vi "Read Loop order.vi"(11 "Toggle 8 in":refnum<class "Toggle 8.lvclass">) -> (2 "Loop order":bool, 3 "Toggle 8 out":refnum<class "Toggle 8.lvclass">)   [LabVIEW 2020, in "Toggle 8.lvclass"]
uses:
  Toggle 8.lvclass
  Toggle 8.lvclass/Toggle 8.ctl
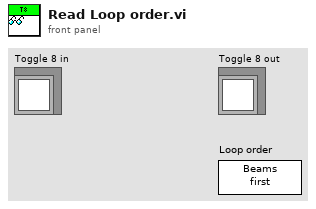
[diagram p1: front panel]
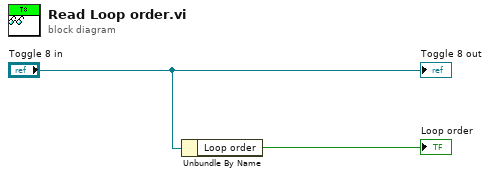
[diagram p0: block diagram]
diagram:
  n1 = Unbundle By Name("Toggle 8 in") -> ("Loop order"=→"Loop order":bool)
  "Toggle 8 out" <- "Toggle 8 in"
